vi "aggregator - t.vi"(4 "complex?":bool=TRUE, 6 "first time":bool=TRUE, 7 "requested size":i32=10, 11 "number":cdb) -> (3 "Array":cdb[](array[numeric]))   [LabVIEW 2012]
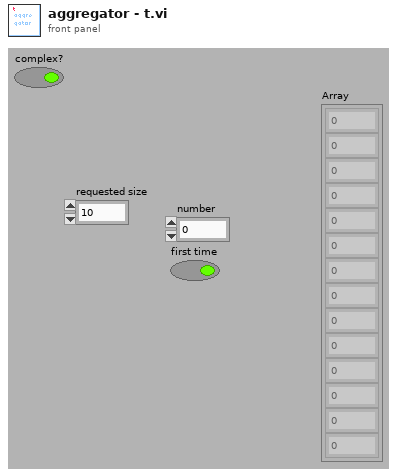
[diagram p1: front panel]
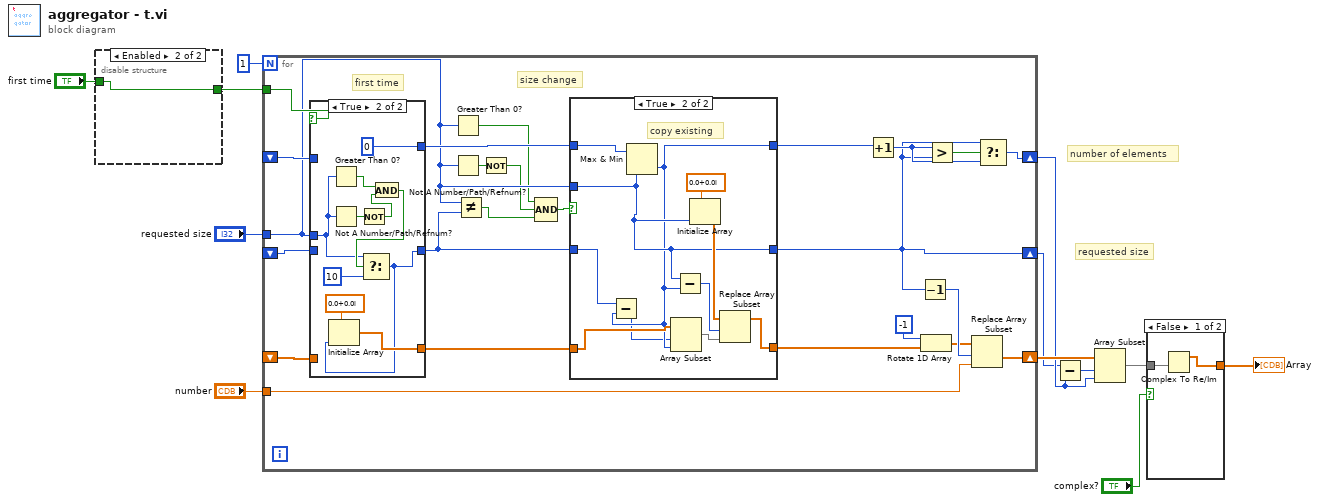
[diagram p0: block diagram]
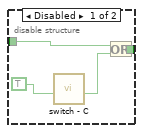
[diagram p3: hidden frame]
diagram:
  # "requested size"
  # "number of elements"
  n1 = disable-structure shown="Enabled" {
    disable-tunnel: "first time" -> [w15 w17]
    disable-tunnel: [w13 w17] -> w4
    frame Disabled {
      n2 = call "switch - C.vi"("switch"=TRUE) -> ("result"=w14:bool)  [unwired: 10 in]
      n3 = Or(x=w15, y=w14) -> (x .or. y?=w13:bool)
    }
    frame Enabled {
    }
  }
  n4 = for {
    N: 1 -> [_]
    tunnel: w4 -> [w32]
    shift-right: [w34] -> w7
    shift-left: _ -> [w31]
    tunnel: "requested size" -> [w23]
    tunnel: "number" -> [w37]
    shift-right: [w33] -> w9
    shift-left: _ -> [w39]
    shift-right: [w27] -> w6
    shift-left: _ -> [w30]
    # "size change"
    # "first time"
    n5 = case shown="True" w32 {
      tunnel: w39 -> [w57 _]
      tunnel: [w57 w66] -> w25
      tunnel: [w58 0] -> w28
      tunnel: [w56 w59] -> w24
      tunnel: w23 -> [_ w61]
      tunnel: w31 -> [w58 _]
      tunnel: w30 -> [w56 _]
      frame False {
      }
      frame True {
        n6 = Greater Than 0?(x=w61) -> (x > 0?=w63:bool)
        n7 = Not A Number/Path/Refnum?(number/path/refnum=w61) -> (NaN/Path/Refnum?=w65:bool)
        n8 = Not(x=w65) -> (.not. x?=w64:bool)
        n9 = And(x=w63, y=w64) -> (x .and. y?=w62:bool)
        n10 = Select(t=w61, s=w62, f=10) -> (s? t:f=w59:i32)
        n11 = Initialize Array(cdb 0.0+0.0i, w59) -> (w66:cdb[])
      }
    }
    n12 = Greater Than 0?(x=w23) -> (x > 0?=w21:bool)
    n13 = Not A Number/Path/Refnum?(number/path/refnum=w23) -> (NaN/Path/Refnum?=w22:bool)
    n14 = Not Equal?(x=w23, y=w24) -> (x != y?=w19:bool)
    n15 = Not(x=w22) -> (.not. x?=w20:bool)
    n16 = Compound Arithmetic op=AND(w21, w20, w19) -> (w18:bool)
    n17 = case shown="True" w18 {
      tunnel: [w44 w47] -> w29
      tunnel: w28 -> [w44 w54]
      tunnel: [w43 w52] -> w27
      tunnel: w24 -> [w43 w46]
      tunnel: [w42 w50] -> w26
      tunnel: w25 -> [w42 w49]
      tunnel: w23 -> [_ w52]
      frame False {
      }
      frame True {
        # "copy existing"
        n18 = Max & Min(x=w54, y=w52) -> (min(x,y)=w47:i32)  [unwired: 1 out]
        n19 = Subtract(x=w46, y=w47) -> (x-y=w45:i32)
        n20 = Array Subset(array=w49, index=w45, length=w47) -> (w48:cdb[])
        n21 = Subtract(x=w52, y=w47) -> (x-y=w51:i32)
        n22 = Initialize Array(cdb 0.0+0.0i, w52) -> (w53:cdb[])
        n23 = Replace Array Subset(array=w53, new element=w48, index=w51) -> (w50:cdb[])
      }
    }
    n24 = Increment(x=w29) -> (x+1=w40:i32)
    n25 = Decrement(x=w27) -> (x-1=w36:i32)
    n26 = Rotate 1D Array(1:w26, 2:-1 ("n")) -> (0:w35:cdb[])
    n27 = Greater?(x=w40, y=w27) -> (0:w41:bool)
    n28 = Replace Array Subset(array=w35, new element=w37, index=w36) -> (w33:cdb[])
    n29 = Select(t=w27, s=w41, f=w40) -> (s? t:f=w34:i32)
  }
  n30 = Subtract(x=w6, y=w7) -> (x-y=w8:i32)
  n31 = Array Subset(array=w9, index=w8, length=w7) -> (w1:cdb[])
  n32 = case shown="False" "complex?" {
    tunnel: [w69 w71] -> w2
    tunnel: w1 -> [w70 w71]
    frame False {
      n33 = Complex To Re/Im(x + iy=w70) -> (x=w69:dbl[])  [unwired: 1 out]
    }
    frame True {
    }
  }
  "Array" <- w2
